vi "PH_Sequencer_Watch.PC calc Synchrolock.vi"(0 "i ref in":refnum<vi>, 5 "error in":errorcluster) -> (14 "i ref out":refnum<vi>, 19 "error out":errorcluster)   [LabVIEW 2014, in "PH_Sequencer_Watch.lvlib"]
doc: "This VI indicates the status of the fs Synchrolock if it is of interest."
uses:
  PH_Sequencer_Watch.lvlib
  PH_Beamline_Chief/PH_Beamline_Chief.Section.ctl
  PH_Basics/PH_Common/PH_Common.lvlib
  PH_Beamline_Chief/PH_Beamline_Chief.lvlib
  PH_BeamlineInformation/PH_BeamlineInformation.lvlib
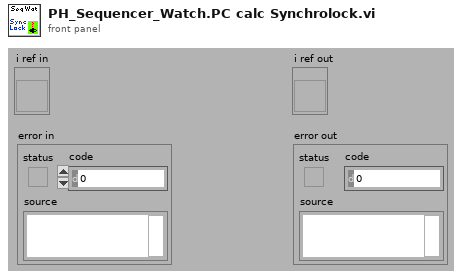
[diagram p1: front panel]
types:
  T1 = typedef "PH_Beamline_Chief.lvlib/PH_Beamline_Chief.Section.ctl" = enum16{"None", "YLF", "fs", "fs-YLF", "ns", "PA-Input", "PA-Undelay", "PA-Delay", "PA-before-Bypass", "PA", "PA-Bypass", "PA-Exit", "PA-LL", "LL", "PA-MA", "MA-Exit", "MA-Z6", "Z6", "MA-LB", "LB-TB2", "LB-TB3"}
  T2 = typedef "PH_Sequencer_Watch.lvlib/PH_Sequencer_Watch.i attribute.ctl" = cluster{"GUI Refs":cluster{"Shot ID":refnum<vi>, "Sequencer SM State":refnum<vi>, "Remaining Time":refnum<vi>, "PHELIX_Timing_T2":refnum<vi>, "T2-Unit-Dummy":refnum<vi>, "fs_Synchrolock_Watch":refnum<vi>, "Experiment_Vacuum_Control_Experiment":refnum<vi>}, "Status Synchrolock":T3, "Exp - Pressure":dbl, "Exp - Limit":dbl, "Heads":T4[], "Refs BooleanState":refnum<vi>[]}
  T3 = typedef "PH_StatusHandler.lvlib/PH_StatusHandler.Status.ctl" = i16
  T4 = typedef "PH_Sequencer_Watch.lvlib/PH_Sequencer_Watch.Head Information.ctl" = cluster{"Ref Volt":refnum<vi>, "PU":T5}
  T5 = typedef "PH_PP_Common.lvlib/PH_PP_Common.PUs.ctl" = enum16{"no Info", "PA-19mm-1", "PA-19mm-2", "PA-45mm-PILC", "PA-45mm-MAIN", "MA-PU-1", "MA-PU-2", "MA-PU-3", "MA-PU-4", "MA-PU-5", "MA-PU-6", "MA-FR", "MA-PILC", "PA-45mm-DP"}
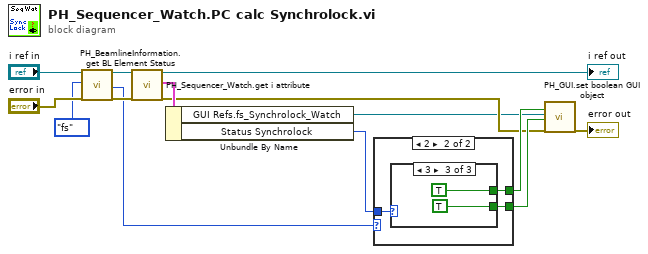
[diagram p0: block diagram]
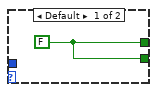
[diagram p2: hidden frame]
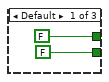
[diagram p3: hidden frame]
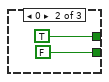
[diagram p4: hidden frame]
diagram:
  n1 = call "PH_BeamlineInformation.get BL Element Status.vi"("VI in"="i ref in", "Beamline Element"=PH_Beamline_Chief.Section."fs" ("Beamline Section"), "error in (no error)"="error in") -> ("VI out"=w3:refnum<vi>, "Status"=w1:i32, "error out"=w5:errorcluster)  [unwired: 14 in]
  n2 = call "PH_Sequencer_Watch.get i attribute.vi"("i ref in"=w3, "error in (no error)"=w5) -> ("i ref out"=→"i ref out":refnum<vi>, "i attribute"=w13:T2, "error out"=w8:errorcluster)  [unwired: 15 in]
  n3 = Unbundle By Name(w13) -> ("GUI Refs.fs_Synchrolock_Watch"=w6:refnum<vi>, "Status Synchrolock"=w12:T3)
  n4 = case shown="2" w1 {
    tunnel: w12 -> [_ w18]
    tunnel: [w15 w17] -> w11
    tunnel: [w15 w16] -> w10
    frame Default {
      w15 = FALSE
    }
    frame 2 {
      n5 = case shown="3" w18 {
        tunnel: [FALSE TRUE TRUE] -> w17
        tunnel: [FALSE FALSE TRUE] -> w16
        frame Default {
        }
        frame 0 {
        }
        frame 3 {
        }
      }
    }
  }
  n6 = call "PH_GUI.set boolean GUI object.vi"("Visible (true)"=w11, "Boolean Knob GUI Ref"=w6, "Value"=w10, "error in (no error)"=w8) -> ("error out"=→"error out":errorcluster)  [unwired: 15 in]
